vi "PolyFit-60to-90_1.vi"(11 "Voltage":dbl) -> (3 "Angle":dbl)   [LabVIEW 2022 SP3]
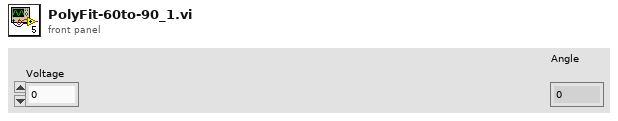
[diagram p1: front panel]
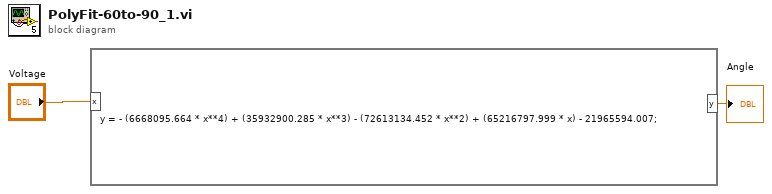
[diagram p0: block diagram]
diagram:
  n1 = formula code="y = - (6668095.664 * x**4) + (35932900.285 * x**3) - (72613134.452 * x**2) + (65216797.999 * x) - 21965594.007;"("x"="Voltage") -> ("y"=→"Angle":dbl)
